vi "Initialize Front Panel.vi"(8 "error in (no error)":errorcluster, 11 "ExampleViewManager in":refnum<class "ExampleViewManager.lvclass">) -> (0 "error out":errorcluster, 3 "ExampleViewManager out":refnum<class "ExampleViewManager.lvclass">)   [LabVIEW 2017, in "MVA Example.lvlib" / "ExampleViewManager.lvclass"]
doc: "<License>\nCopyright © 2017 Composed Systems, LLC | All rights reserved\nwww.composed.io\n\nAuthor: Ethan Stern <ethan.stern@composed.io>\n\nThis software is provided \"AS IS\" WITHOUT WARRANTIES, either express or implied, AND IS FOR EDUCATIONAL PURPOSES ONLY.\n</License>MVA Framework 1.6.0.31\nEthan Stern - Composed Systems\nCopyright (c) 2018, Composed Systems"
uses:
  ExampleViewManager.lvclass
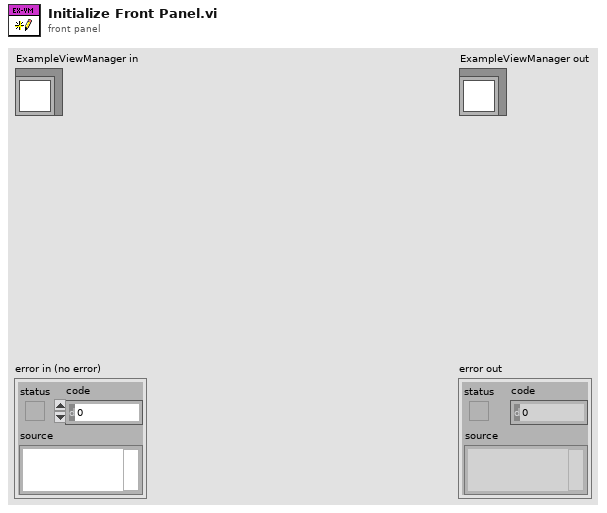
[diagram p1: front panel]
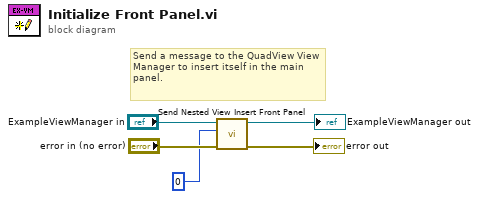
[diagram p0: block diagram]
diagram:
  # "Send a message to the QuadView View Manager to insert itself in the main panel."
  n1 = call "Send Nested View Insert Front Panel.vi"("error in (no error)"="error in (no error)", "View Index"=0, "ExampleViewManager in"="ExampleViewManager in") -> ("error out"=→"error out":errorcluster, "ExampleViewManager out"=→"ExampleViewManager out":refnum<class "ExampleViewManager.lvclass">)  [unwired: 7 in]
